vi "Public Async Request.vi"(6 "Callback":refnum<class "Callback.lvclass">, 8 "error in (no error)":errorcluster, 9 "Request Message Data":variant, 10 "Request Message":string, 11 "Mock Process in":refnum<class "Mock Process.lvclass">) -> (0 "error out":errorcluster, 3 "Mock Process out":refnum<class "Mock Process.lvclass">)   [LabVIEW 2020, in "Mock Process.lvclass"]
uses:
  Mock Process.lvclass
  C:/git/astemes-triarc-framework/source/Framework/Process/Process.lvclass
  Framework/Callback/Callback.lvclass
  Framework/Process/Process.lvclass/Process.ctl
  Framework/Process/Private/SubVIs/Handle Debug Data.vi
  Framework/Logging/Log Debug.vi
  <vilib>/AdvancedString/1D String Array to Delimited String.vi
  <vilib>/Utility/High Resolution Relative Seconds.vi
  Framework/Process/Process.lvclass
  C:/git/astemes-triarc-framework/source/Framework/Logging/Logging.lvclass
  Framework/Process/Public/Read Name.vi
  Framework/Logging/Logging.lvclass
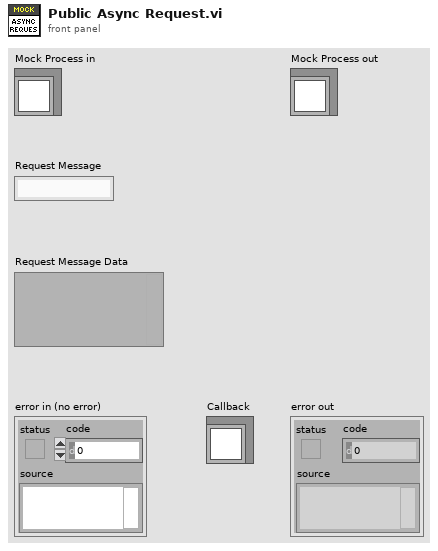
[diagram p1: front panel]
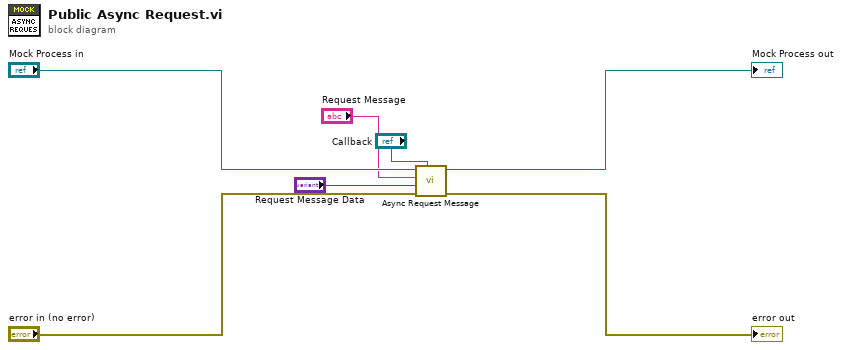
[diagram p0: block diagram]
diagram:
  n1 = call "Async Request Message.vi"("Callback"="Callback", "error in (no error)"="error in (no error)", "Request Message Data"="Request Message Data", "Request Message"="Request Message", "Process In"="Mock Process in") -> ("error out"=→"error out":errorcluster, "Process Out"=→"Mock Process out":refnum<class "Mock Process.lvclass">)  [unwired: 3 in]
